vi "Close.vi"(8 "error in (no error)":errorcluster, 11 "VISA TCP in":refnum<class "VISA TCP.lvclass">) -> (0 "error out":errorcluster, 3 "VISA TCP out":refnum<class "VISA TCP.lvclass">)   [LabVIEW 2021, in "Sockets.lvlib" / "VISA TCP.lvclass"]
doc: "Closes the socket connection.\nWebSockets 2.0.1.40\nSam Sharp - MediaMongrels Ltd\nCopyright (c) 2019, MediaMongrels Ltd"
uses:
  VISA TCP.lvclass
  VISA TCP.lvclass/VISA TCP.ctl
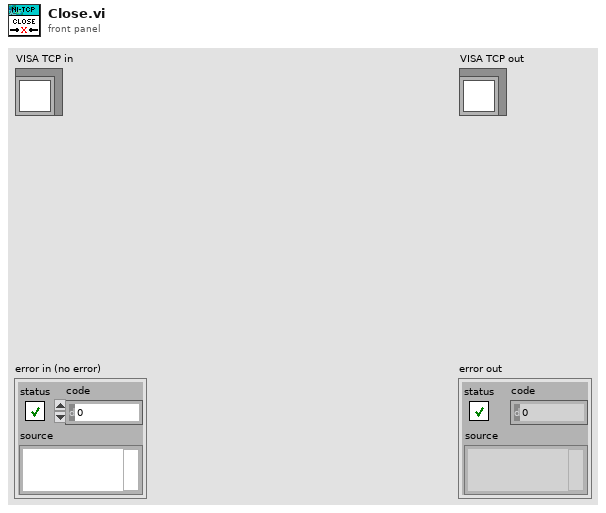
[diagram p1: front panel]
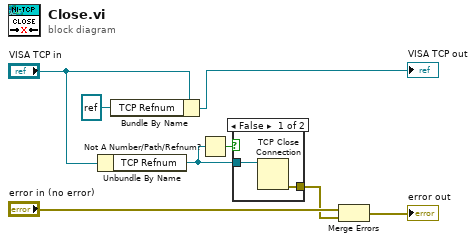
[diagram p0: block diagram]
diagram:
  n1 = Unbundle By Name("VISA TCP in") -> ("TCP Refnum"=w2:refnum<k5>)
  n2 = Bundle By Name(cluster="VISA TCP in", "TCP Refnum"=refnum<k5> refnum) -> (→"VISA TCP out":refnum<class "VISA TCP.lvclass">)
  n3 = Not A Number/Path/Refnum?(number/path/refnum=w2) -> (NaN/Path/Refnum?=w1:bool)
  n4 = case shown="False" w1 {
    tunnel: w2 -> [w10 _]
    tunnel: [w9 _] -> w7
    frame False {
      n5 = TCP Close Connection(connection ID=w10) -> (error out=w9:errorcluster)  [unwired: 2 in, 1 out]
    }
    frame True {
    }
  }
  n6 = Merge Errors("error in (no error)", w7) -> (→"error out":errorcluster)
